vi "Is Readout Flipped By Amplifier.vi"(8 "error in (no error)":errorcluster, 10 "iFlipped":i32, 11 "iAmplifier":i32) -> (0 "error out":errorcluster, 2 "iFlipped out":i32, 3 "function return":u32)   [LabVIEW 2014, in "atmcd32d.lvlib"]
doc: "unsigned int WINAPI IsReadoutFlippedByAmplifier(int iAmplifier, int * iFlipped);"
uses:
  atmcd32d.lvlib
  atmcd32d.dll
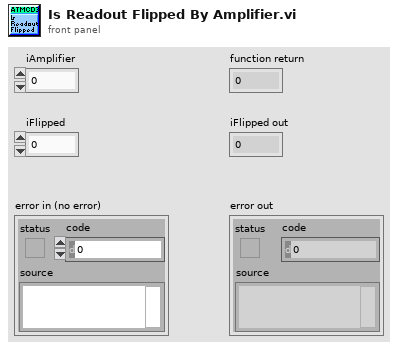
[diagram p1: front panel]
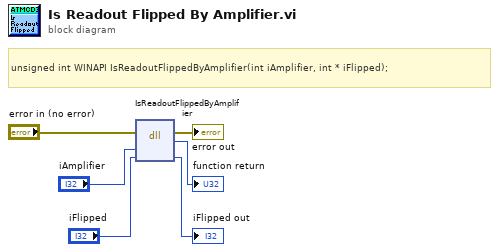
[diagram p0: block diagram]
diagram:
  # "unsigned int WINAPI IsReadoutFlippedByAmplifier(int iAmplifier, int * iFlipped);"
  n1 = dll-call lib="C:/Users/Bakir/Documents/Lambda2-Testing/lib/Andorlib/atmcd32d.*" fn="IsReadoutFlippedByAmplifier"(error in="error in (no error)", "iAmplifier"="iAmplifier", "iFlipped"="iFlipped") -> (error out=→"error out":errorcluster, →"function return":u32, "iFlipped"=→"iFlipped out":i32)  [unwired: 3 in, 1 out]
